vi "sensor_test.vi"() -> ()   [LabVIEW 2020]
panel:
  in  "stop":bool
  out "TCI2":dbl
  out "SGI2":dbl format="%#_6f"
  out "TCI1":dbl
  out "SGI1":dbl format="%#_6f"
  out "TCI0":dbl
  out "SGI0":dbl format="%#_6f"
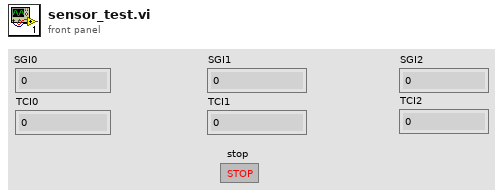
[diagram p1: front panel]
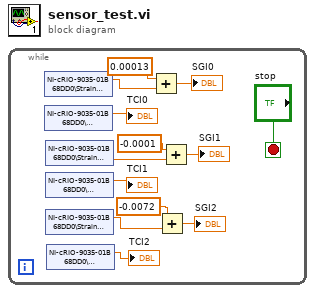
[diagram p0: block diagram]
diagram:
  n1 = while {
    stop <- "stop" stop-if-true
    n2 = shared-variable "NI-cRIO-9035-01B68DD0\\Strain Gauge\\SGI0"() -> (w7:dbl)  [unwired: 1 in, 1 out]
    n3 = shared-variable "NI-cRIO-9035-01B68DD0\\Thermocouple\\TCI0"() -> (→"TCI0":dbl)  [unwired: 1 in, 1 out]
    n4 = shared-variable "NI-cRIO-9035-01B68DD0\\Strain Gauge\\SGI1"() -> (w3:dbl)  [unwired: 1 in, 1 out]
    n5 = shared-variable "NI-cRIO-9035-01B68DD0\\Thermocouple\\TCI1"() -> (→"TCI1":dbl)  [unwired: 1 in, 1 out]
    n6 = shared-variable "NI-cRIO-9035-01B68DD0\\Strain Gauge\\SGI2"() -> (w6:dbl)  [unwired: 1 in, 1 out]
    n7 = shared-variable "NI-cRIO-9035-01B68DD0\\Thermocouple\\TCI2"() -> (→"TCI2":dbl)  [unwired: 1 in, 1 out]
    n8 = Add(x=0.00013, y=w7) -> (x+y=→"SGI0":dbl)
    n9 = Add(x=-0.0072, y=w6) -> (x+y=→"SGI2":dbl)
    n10 = Add(x=-0.0001, y=w3) -> (x+y=→"SGI1":dbl)
  }
